vi "声音信号采集.vi"() -> ()   [LabVIEW 2018]
uses:
  <vilib>/sound2/lvsound2.llb/Sampling Mode.ctl
  <vilib>/sound2/lvsound2.llb/Sound Data Format.ctl
  <vilib>/sound2/lvsound2.llb/Sound Input Read (DBL).vi
panel:
  in  "停止按钮":bool
  in  "空白按钮":bool
  out "error out":errorcluster caption="错误输出"
  in  "sound format":T1={"sample rate (S/s)"=22050.0, "number of channels"=2, "bits per sample"=16} caption="声音格式"
  in  "device ID":u32 caption="设备ID"
  in  "sample mode":T2=1 caption="采样模式" items=["有限采样", "连续采样"]
  out "语音信号时域波形":waveform(dbl)[](graph)
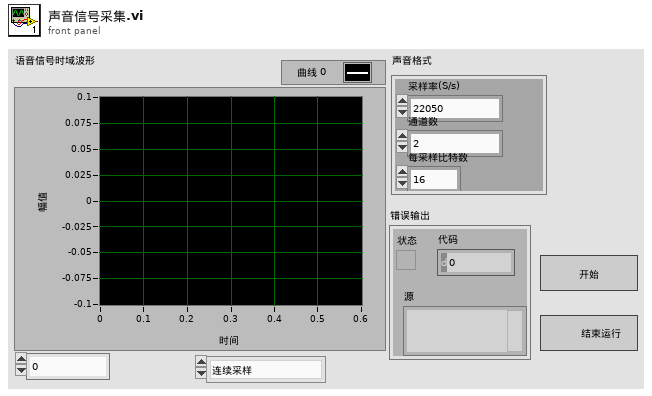
[diagram p1: front panel]
types:
  T1 = typedef "Sound Data Format.ctl" = cluster{"sample rate (S/s)":dbl, "number of channels":i32, "bits per sample":i32}
  T2 = typedef "Sampling Mode.ctl" = i32
  T3 = typedef "Sound Input Task ID.ctl" = u32
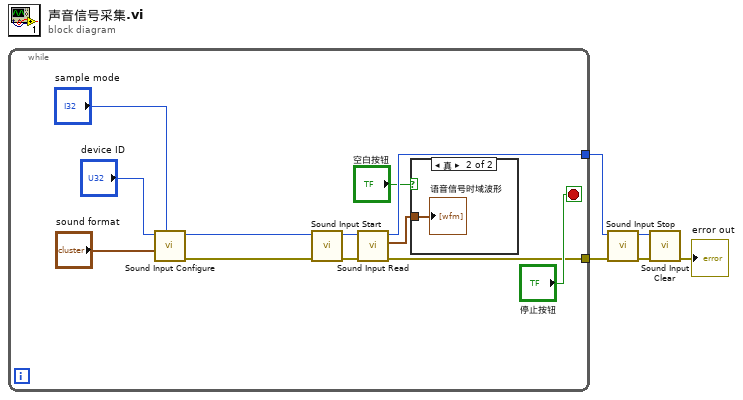
[diagram p0: block diagram]
diagram:
  n1 = while {
    tunnel: [w13] -> w4
    tunnel: [w10] -> w3
    stop <- "停止按钮" stop-if-true
    n2 = call <vilib>:"Sound Input Configure.vi"("sample mode"="sample mode", "sound format"="sound format", "device ID"="device ID") -> ("error out"=w16:errorcluster, "task ID"=w6:T3)  [unwired: 7 in]
    n3 = call <vilib>:"Sound Input Start.vi"("error in (no error)"=w16, "task ID"=w6) -> ("error out"=w14:errorcluster, "task ID out"=w15:T3)  [unwired: 8 in]
    n4 = call-poly <vilib>:"Sound Input Read.vi"("error in (no error)"=w14, "task ID"=w15) -> ("error out"=w10:errorcluster, "data"=w7:waveform(dbl)[], "task ID out"=w13:T3)  [unwired: 7 in]
    n5 = case shown="真" "空白按钮" {
      tunnel: w7 -> [_ w18]
      frame False {
      }
      frame True {
        "语音信号时域波形" <- w18
      }
    }
  }
  n6 = call <vilib>:"Sound Input Stop.vi"("error in (no error)"=w3, "task ID"=w4) -> ("error out"=w1:errorcluster, "task ID out"=w2:T3)  [unwired: 8 in]
  n7 = call <vilib>:"Sound Input Clear.vi"("error in (no error)"=w1, "task ID"=w2) -> ("error out"=→"error out":errorcluster)  [unwired: 9 in]
